vi "Config Aout Limit.vi"(6 "Lower Loss (-10.5 V)":dbl=-10.5 min=-10.5 max=10.5 format="%#_6f", 7 "Upper Capacitance (10.5 V)":dbl=10.5 min=-10.5 max=10.5 format="%#_6f", 8 "error in":errorcluster, 9 "Lower Capacitance (-10.5 V)":dbl=-10.5 min=-10.5 max=10.5 format="%#_6f", 10 "Upper Loss (10.5 V)":dbl=10.5 min=-10.5 max=10.5 format="%#_6f", 11 "VISA resource name":refnum<visa-resource-name>) -> (0 "error out":errorcluster, 3 "VISA resource name out":refnum<visa-resource-name>)   [LabVIEW 2017, in "Andeen-Hagerling 2700.lvlib"]
doc: "This VI sets the upper and lower protection limits, respectively, of the capacitance and loss channel output voltages in volts. These protection limits apply only to voltage levels produced by the deviation subsystem. They do not limit the output derived from internal bias voltage sources."
uses:
  Andeen-Hagerling 2700.lvlib
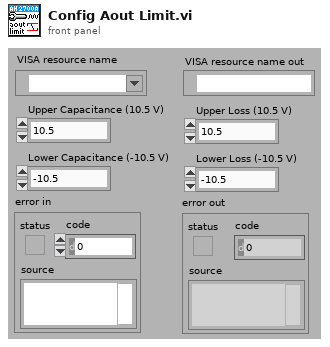
[diagram p1: front panel]
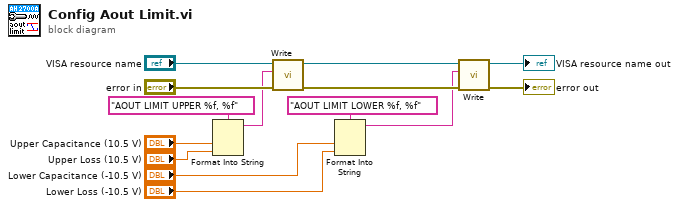
[diagram p0: block diagram]
diagram:
  n1 = Format Into String(format string="AOUT LIMIT UPPER %f, %f", "Upper Capacitance (10.5 V)", "Upper Loss (10.5 V)") -> (resulting string=w9:string)  [unwired: 2 in, 1 out]
  n2 = call "Write.vi"("error in"="error in", "command"=w9, "VISA resource name"="VISA resource name") -> ("error out"=w6:errorcluster, "VISA resource name out"=w8:refnum<visa-resource-name>)  [unwired: 7 in]
  n3 = Format Into String(format string="AOUT LIMIT LOWER %f, %f", "Lower Capacitance (-10.5 V)", "Lower Loss (-10.5 V)") -> (resulting string=w2:string)  [unwired: 2 in, 1 out]
  n4 = call "Write.vi"("error in"=w6, "command"=w2, "VISA resource name"=w8) -> ("error out"=→"error out":errorcluster, "VISA resource name out"=→"VISA resource name out":refnum<visa-resource-name>)  [unwired: 7 in]
